vi "Read.vi"(8 "error in (no error)":errorcluster, 11 "UI VISA Terminal in":refnum<class "UI VISA Terminal.lvclass">) -> (0 "error out":errorcluster, 3 "UI VISA Terminal out":refnum<class "UI VISA Terminal.lvclass">)   [LabVIEW 2025, in "UI VISA Terminal.lvlib" / "UI VISA Terminal.lvclass"]
uses:
  UI VISA Terminal.lvclass
  UI VISA Terminal.lvclass/UI VISA Terminal.ctl
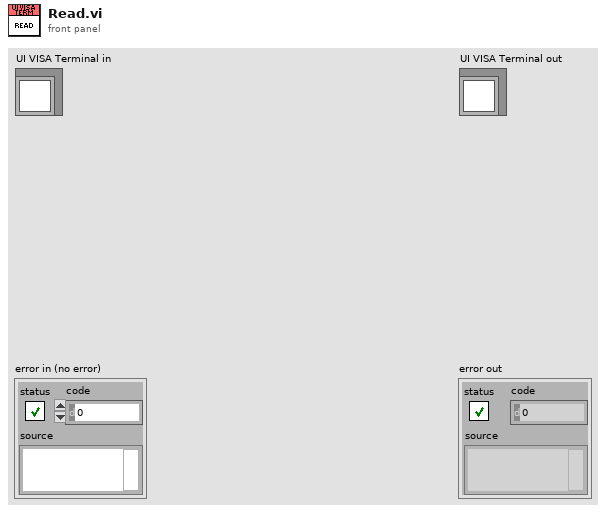
[diagram p1: front panel]
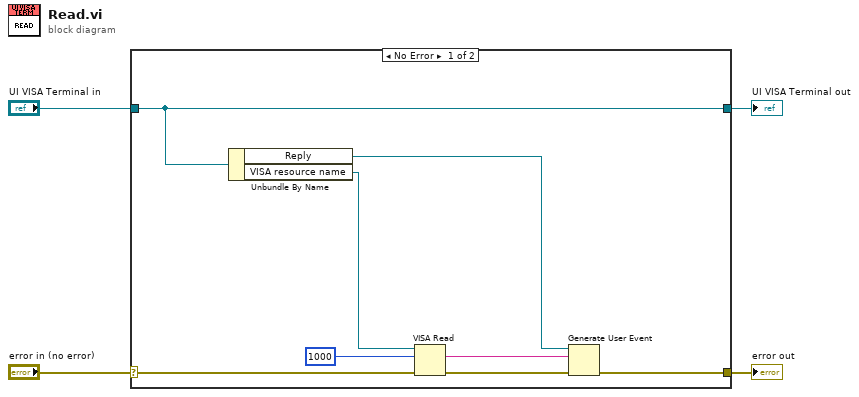
[diagram p0: block diagram]
diagram:
  n1 = case shown="No Error" "error in (no error)" {
    selector: "error in (no error)" -> [w12 w14]
    tunnel: [w7 w14] -> w3
    tunnel: [w10 w13] -> w1
    tunnel: "UI VISA Terminal in" -> [w10 w13]
    frame No Error {
      n2 = Unbundle By Name(w10) -> ("Reply"=w6:refnum<user-event>, "VISA resource name"=w9:refnum<visa-resource-name>)
      n3 = VISA Read(VISA resource name=w9, byte count=u32 1000, error in (no error)=w12) -> (read buffer=w5:string, error out=w11:errorcluster)  [unwired: 2 out]
      n4 = Generate User Event(user event=w6, event data cluster=w5, error in=w11) -> (error out=w7:errorcluster)  [unwired: 1 in, 1 out]
    }
    frame Error {
    }
  }
  "error out" <- w3
  "UI VISA Terminal out" <- w1
